vi "RIOTargetUI.vi"() -> ()   [LabVIEW 2014, in "RIO Target.lvclass"]
doc: "UI that will be called when the node is selected."
uses:
  RIO Target/RIO Target.lvclass
  <vilib>/NI/Configuration Framework/Node/NodeRef.ctl
  <vilib>/NI/Configuration Framework/Node/NISE_CEF_Node.lvclass
  <vilib>/NI/AMC/Message Queue.ctl
  <vilib>/NI/AMC/Message.ctl
  <vilib>/NI/Tools/Keyed Array/KeyedArray.ctl
  <vilib>/NI/Configuration Framework/Node/UserEventRef.ctl
  <vilib>/NI/Configuration Framework/Controls/EventCluster.ctl
  RIO Target/RIO Target.lvclass/RIO Target.ctl
  RIO Target Configuration/RIO Target Configuration.lvclass/RIO Target Configuration.ctl
  RIO Target Configuration/RIO Target Configuration.lvclass
  <vilib>/NI/Configuration Framework/serializable configuration/NISE_CEF_serializable configuration.lvclass
  <vilib>/NI/Tools/Keyed Array/Tools_KeyedArray.lvlib
  <vilib>/NI/AMC/AMC.lvlib
  <vilib>/NI/Configuration Framework/NISE_CEF_TreeControl.lvlib
panel:
  in  "CLIP XML Path":path
  in  "Use Custom CLIP?":bool
  out "Number of Channels":u32
  out "Number of Devices":u32
  out "Number of Buses":u32
  out "Channels per Device":string[][](table)
  in  "Target Destination VI":path
  in  "Replace Default Destination VI?":bool
  in  "Target Project Path":path
  in  "Comments":string
  in  "Alias":string
  in  "user event":T1
  in  "main queue":T2
  in  "node ref":T3
  # "Settings"
  # "Target Destination VI"
  # "CLIP XML Path"
  # "Target Summary"
  # "Number of Buses"
  # "Number of Devices"
  # "Number of Channels"
  # "Channels per Device"
  # "Target Project Path"
  # "Comments"
  # "Alias"
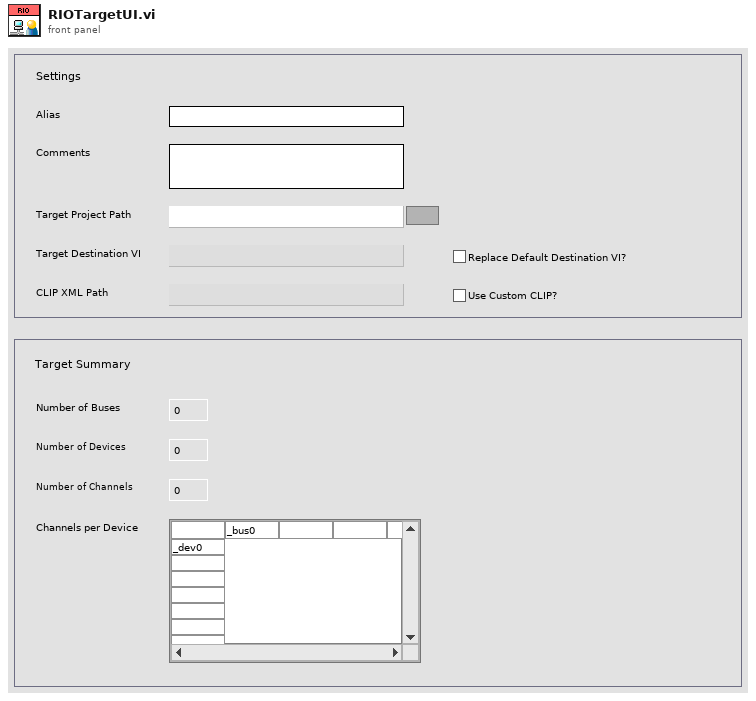
[diagram p1: front panel]
types:
  T1 = typedef "NISE_CEF_Node.lvclass/UserEventRef.ctl" = refnum<user-event>
  T2 = typedef "AMC.lvlib/Message Queue.ctl" = refnum<queue>
  T3 = typedef "NISE_CEF_Node.lvclass/NodeRef.ctl" = refnum<data-value>
  T4 = typedef "RIO Target.lvclass/UI Configuration.ctl" = cluster{"Destination VI":path, "Target Project Path":path, "CLIP XML Path":path, "Alias":string, "Comments":string, "Replace Default VI?":bool, "Use Custom CLIP?":bool}
  T5 = enum8{"Enabled", "Disabled", "Disabled and Grayed Out"}
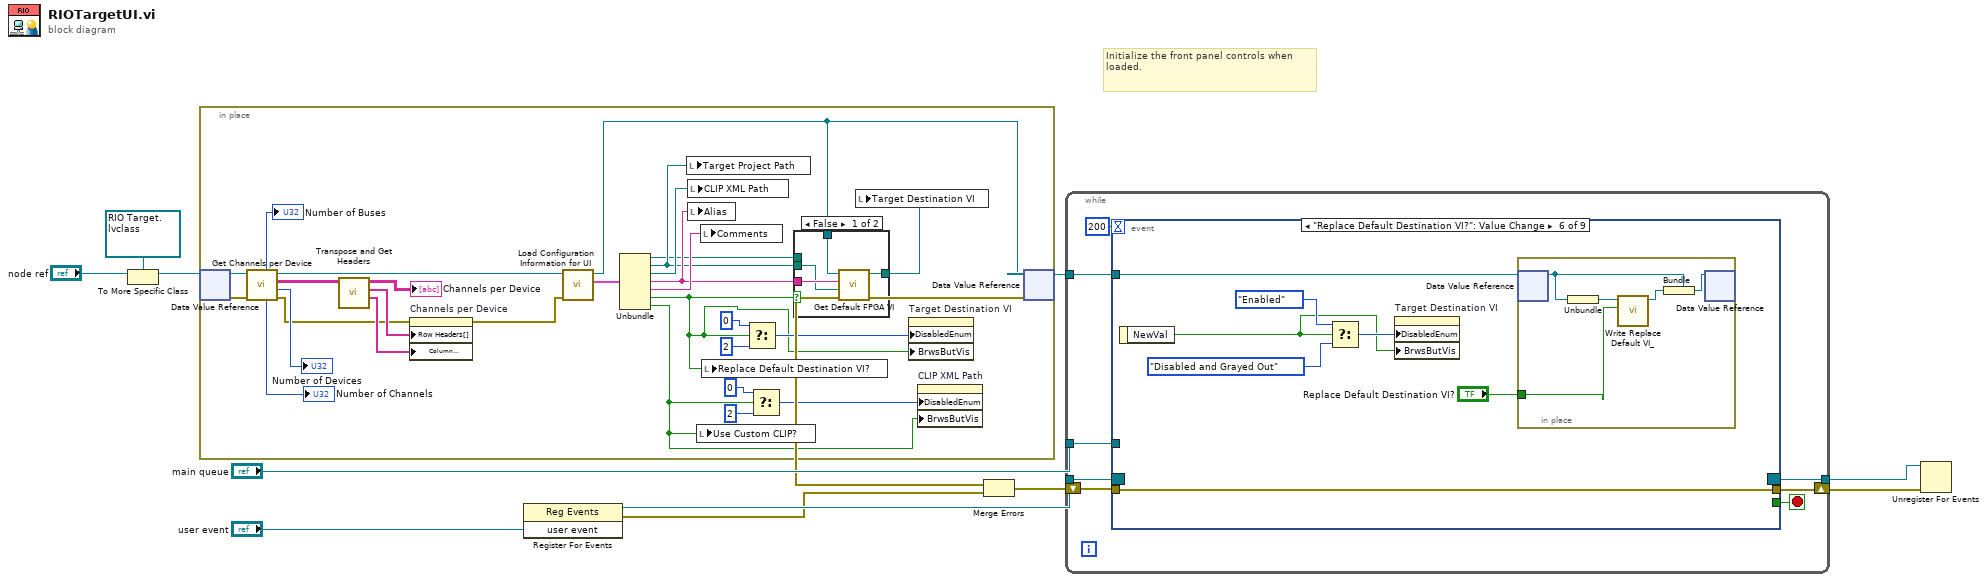
[diagram p0: block diagram]
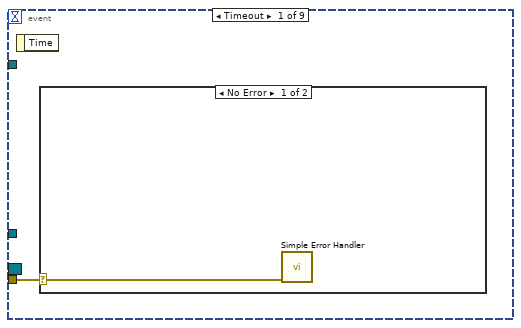
[diagram p2: hidden frame]
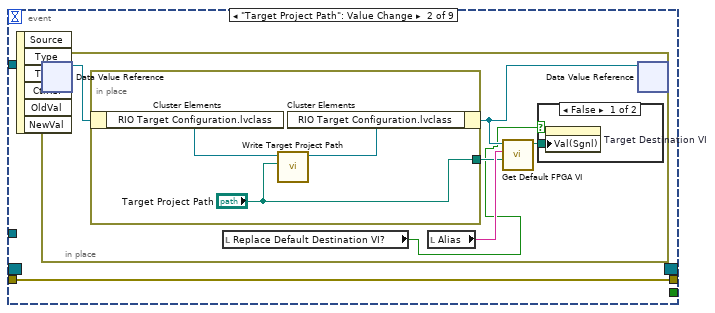
[diagram p4: hidden frame]
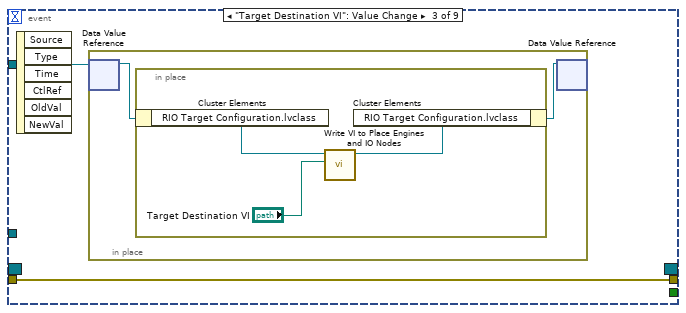
[diagram p6: hidden frame]
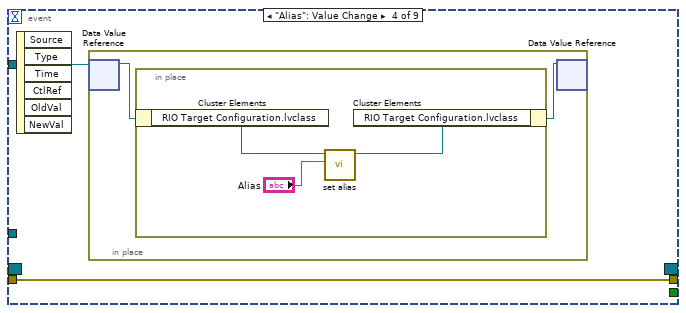
[diagram p7: hidden frame]
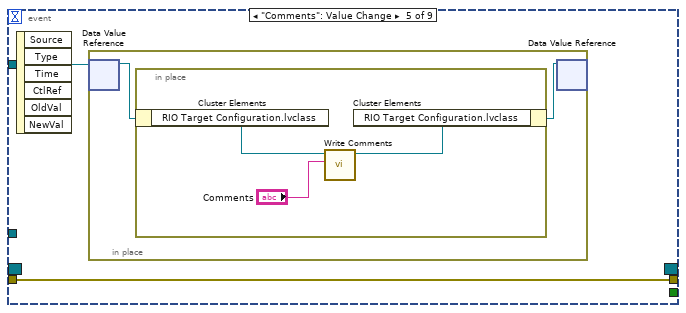
[diagram p8: hidden frame]
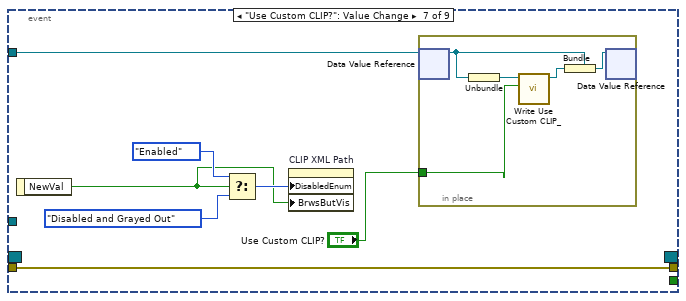
[diagram p9: hidden frame]
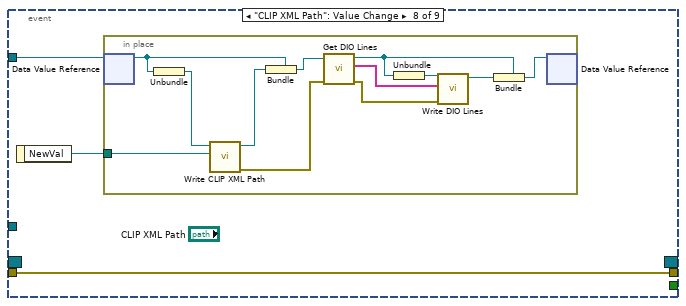
[diagram p10: hidden frame]
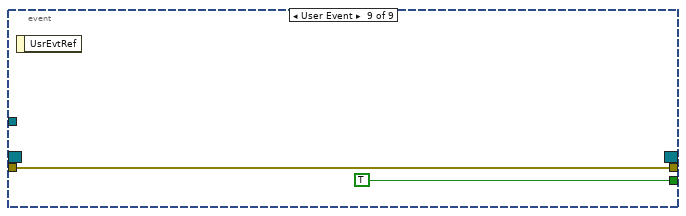
[diagram p11: hidden frame]
diagram:
  # "Initialize the front panel controls when loaded."
  n1 = To More Specific Class(target class=refnum<data-value> refnum ("data value reference"), reference="node ref") -> (specific class reference=w2:refnum<data-value>)  [unwired: 1 in, 1 out]
  n2 = in-place {
    n3 = in-place-dvr #1(w2) -> (w40:refnum<class "RIO Target.lvclass">, w39:errorcluster)
    n4 = call "Get Channels per Device.vi"("error in (no error)"=w39, "RIO Target in"=w40) -> ("error out"=w31:errorcluster, "Number of Devices"=→"Number of Devices":i32, "Channels per Device"=w35:string[][], "RIO Target out"=w30:refnum<class "RIO Target.lvclass">, "Number of Channels"=→"Number of Channels":u32, "Number of Buses"=→"Number of Buses":i32)  [unwired: 4 in]
    n5 = call "Transpose and Get Headers.vi"("Channels per Device'"=w35) -> ("Column Headers"=w32:string[], "Row Headers"=w33:string[], "Channels per Device"=→"Channels per Device":string[][])  [unwired: 8 in]
    n6 = property on="Channels per Device" class="Tbl (strict)"(error in=w31, "Row Headers[]"=w33, "Column Headers[]"=w32) -> (error out=w29:errorcluster)  [unwired: 1 in, 1 out]
    n7 = call "Load Configuration Information for UI.vi"("error in (no error)"=w29, "node in"=w30) -> ("UI Configuration"=w28:T4, "node out"=w15:refnum<class "RIO Target.lvclass">)  [unwired: 7 in, 1 out]
    n8 = Unbundle(w28) -> ("Destination VI"=w23:path, "Target Project Path"=w24:path, "CLIP XML Path"=w27:path, "Alias"=w25:string, "Comments"=w26:string, "Replace Default VI?"=w16:bool, "Use Custom CLIP?"=w13:bool)
    n9 = local write "Target Project Path"(w24) -> ()
    n10 = local write "CLIP XML Path"(w27) -> ()
    n11 = local write "Alias"(w25) -> ()
    n12 = local write "Use Custom CLIP?"(w13) -> ()
    n13 = local write "Comments"(w26) -> ()
    n14 = local write "Replace Default Destination VI?"(w16) -> ()
    n15 = Select(t=0, s=w16, f=2) -> (s? t:f=w18:i32)
    n16 = Select(t=0, s=w13, f=2) -> (s? t:f=w17:i32)
    n17 = case shown="False" w16 {
      tunnel: w15 -> [w44 _]
      tunnel: w25 -> [w43 _]
      tunnel: w24 -> [w42 _]
      tunnel: [w41 w45] -> w22
      tunnel: w23 -> [_ w45]
      frame False {
        n18 = call "Get Default FPGA VI.vi"("Target Project Path"=w42, "Alias"=w43, "LabVIEW Object in"=w44) -> ("appended path"=w41:path)  [unwired: 8 in]
      }
      frame True {
      }
    }
    n19 = local write "Target Destination VI"(w22) -> ()
    n20 = property on="Target Destination VI" class="Path"("DisabledEnum"=w18, "BrwsButVis"=w16) -> ()  [unwired: 2 in, 2 out]
    n21 = property on="CLIP XML Path" class="Path"("DisabledEnum"=w17, "BrwsButVis"=w13) -> ()  [unwired: 2 in, 2 out]
    n22 = in-place-dvr #1(w15) -> (w12:refnum<data-value>, w6:errorcluster)
  }
  n23 = register-events("user event") -> (reference out=w9:refnum<event-registration>, error out=w1:errorcluster)  [unwired: 2 in]
  n24 = Merge Errors(w6, w1) -> (w5:errorcluster)
  n25 = while {
    tunnel: w12 -> [w53]
    tunnel: "main queue" -> [w52]
    tunnel: w9 -> [w50]
    tunnel: [w49] -> w8
    shift-right: [w47] -> w7
    shift-left: w5 -> [w46]
    stop <- w48 stop-if-true
    n26 = event shown="[5] \"Replace Default Destination VI?\": Value Change" {
      selector: w50 -> [_ _ _ _ _ _ _ _ _]
      dyn-events: [_ _ _ _ _ _ _ _ _] -> w49
      timeout: 200 -> [_ _ _ _ _ _ _ _ _]
      tunnel: w53 -> [_ w56 w68 w75 w82 w90 w102 w114 _]
      tunnel: w52 -> [_ _ _ _ _ _ _ _ _]
      tunnel: [_ _ _ _ _ _ _ _ TRUE] -> w48
      tunnel: [_ w57 w69 w76 w83 w95 w107 w115 w128] -> w47
      tunnel: w46 -> [w54 w57 w69 w76 w83 w95 w107 w115 w128]
      event Timeout {
        n27 = event-data() -> ()  [unwired: 1 in, 1 out]
        n28 = case shown="No Error" w54 {
          selector: w54 -> [w55 _]
          frame No Error {
            n29 = call <vilib>:"Simple Error Handler.vi"("error in (no error)"=w55) -> ()  [unwired: 4 in, 5 out]
          }
          frame Error {
          }
        }
      }
      event "Target Project Path": Value Change {
        n30 = event-data() -> ()  [unwired: 1 in, 6 out]
        n31 = in-place {
          n32 = in-place-dvr #2(w56) -> (w63:refnum<class "RIO Target.lvclass">)  [unwired: 1 out]
          n33 = in-place {
            in-place-border: ["Target Project Path"] -> w59
            n34 = in-place-cluster #3(w63) -> ("RIO Target Configuration.lvclass"=w67:refnum<class "RIO Target Configuration.lvclass">)
            n35 = call "Write Target Project Path.vi"("Target Project Path"="Target Project Path", "RIO Target Configuration in"=w67) -> ("RIO Target Configuration out"=w66:refnum<class "RIO Target Configuration.lvclass">)  [unwired: 8 in, 1 out]
            n36 = in-place-cluster #3("RIO Target Configuration.lvclass"=w66) -> (w62:refnum<class "RIO Target.lvclass">)
          }
          n37 = local read "Replace Default Destination VI?"() -> (w58:bool)
          n38 = local read "Alias"() -> (w61:string)
          n39 = call "Get Default FPGA VI.vi"("Target Project Path"=w59, "Alias"=w61, "LabVIEW Object in"=w62) -> ("appended path"=w60:path)  [unwired: 8 in]
          n40 = case shown="False" w58 {
            tunnel: w60 -> [w64 _]
            frame False {
              n41 = property on="Target Destination VI" class="Path"("Val(Sgnl)"=w64) -> ()  [unwired: 2 in, 2 out]
            }
            frame True {
            }
          }
          n42 = in-place-dvr #2(w62) -> ()  [unwired: 2 out]
        }
      }
      event "Target Destination VI": Value Change {
        n43 = event-data() -> ()  [unwired: 1 in, 6 out]
        n44 = in-place {
          n45 = in-place-dvr #4(w68) -> (w71:refnum<class "RIO Target.lvclass">)  [unwired: 1 out]
          n46 = in-place {
            n47 = in-place-cluster #5(w71) -> ("RIO Target Configuration.lvclass"=w74:refnum<class "RIO Target Configuration.lvclass">)
            n48 = call "Write VI to Place Engines and IO Nodes.vi"("VI to Place Engines and IO Nodes"="Target Destination VI", "RIO Target Configuration in"=w74) -> ("RIO Target Configuration out"=w73:refnum<class "RIO Target Configuration.lvclass">)  [unwired: 8 in, 1 out]
            n49 = in-place-cluster #5("RIO Target Configuration.lvclass"=w73) -> (w70:refnum<class "RIO Target.lvclass">)
          }
          n50 = in-place-dvr #4(w70) -> ()  [unwired: 2 out]
        }
      }
      event "Alias": Value Change {
        n51 = event-data() -> ()  [unwired: 1 in, 6 out]
        n52 = in-place {
          n53 = in-place-dvr #6(w75) -> (w78:refnum<class "RIO Target.lvclass">)  [unwired: 1 out]
          n54 = in-place {
            n55 = in-place-cluster #7(w78) -> ("RIO Target Configuration.lvclass"=w81:refnum<class "RIO Target Configuration.lvclass">)
            n56 = call <vilib>:"set alias.vi"("alias"="Alias", "configuration in"=w81) -> ("configuration out"=w80:refnum<class "RIO Target Configuration.lvclass">)  [unwired: 8 in, 1 out]
            n57 = in-place-cluster #7("RIO Target Configuration.lvclass"=w80) -> (w77:refnum<class "RIO Target.lvclass">)
          }
          n58 = in-place-dvr #6(w77) -> ()  [unwired: 2 out]
        }
      }
      event "Comments": Value Change {
        n59 = event-data() -> ()  [unwired: 1 in, 6 out]
        n60 = in-place {
          n61 = in-place-dvr #8(w82) -> (w85:refnum<class "RIO Target.lvclass">)  [unwired: 1 out]
          n62 = in-place {
            n63 = in-place-cluster #9(w85) -> ("RIO Target Configuration.lvclass"=w88:refnum<class "RIO Target Configuration.lvclass">)
            n64 = call "Write Comments.vi"("Comments"="Comments", "RIO Target Configuration in"=w88) -> ("RIO Target Configuration out"=w87:refnum<class "RIO Target Configuration.lvclass">)  [unwired: 8 in, 1 out]
            n65 = in-place-cluster #9("RIO Target Configuration.lvclass"=w87) -> (w84:refnum<class "RIO Target.lvclass">)
          }
          n66 = in-place-dvr #8(w84) -> ()  [unwired: 2 out]
        }
      }
      event "Replace Default Destination VI?": Value Change {
        n67 = event-data() -> ("NewVal"=w91:bool)  [unwired: 1 in]
        n68 = Select(t=T5."Enabled" ("Disabled"), s=w91, f=T5."Disabled and Grayed Out" ("Disabled")) -> (s? t:f=w92:T5)
        n69 = property on="Target Destination VI" class="Path"("DisabledEnum"=w92, "BrwsButVis"=w91) -> ()  [unwired: 2 in, 2 out]
        n70 = in-place {
          in-place-border: "Replace Default Destination VI?" -> [w99]
          n71 = in-place-dvr #10(w90) -> (w97:refnum<class "RIO Target.lvclass">)  [unwired: 1 out]
          n72 = Unbundle(w97) -> (w100:refnum<class "RIO Target Configuration.lvclass">)
          n73 = call "Write Replace Default VI_.vi"("Replace Default VI?"=w99, "RIO Target Configuration in"=w100) -> ("RIO Target Configuration out"=w98:refnum<class "RIO Target Configuration.lvclass">)  [unwired: 8 in, 1 out]
          n74 = Bundle(cluster=w97, w98) -> (w96:refnum<class "RIO Target.lvclass">)
          n75 = in-place-dvr #10(w96) -> ()  [unwired: 2 out]
        }
      }
      event "Use Custom CLIP?": Value Change {
        n76 = event-data() -> ("NewVal"=w103:bool)  [unwired: 1 in]
        n77 = Select(t=T5."Enabled" ("Disabled"), s=w103, f=T5."Disabled and Grayed Out" ("Disabled")) -> (s? t:f=w104:T5)
        n78 = property on="CLIP XML Path" class="Path"("DisabledEnum"=w104, "BrwsButVis"=w103) -> ()  [unwired: 2 in, 2 out]
        n79 = in-place {
          in-place-border: "Use Custom CLIP?" -> [w111]
          n80 = in-place-dvr #11(w102) -> (w109:refnum<class "RIO Target.lvclass">)  [unwired: 1 out]
          n81 = Unbundle(w109) -> (w112:refnum<class "RIO Target Configuration.lvclass">)
          n82 = call "Write Use Custom CLIP_.vi"("Use Custom CLIP?"=w111, "RIO Target Configuration in"=w112) -> ("RIO Target Configuration out"=w110:refnum<class "RIO Target Configuration.lvclass">)  [unwired: 8 in, 1 out]
          n83 = Bundle(cluster=w109, w110) -> (w108:refnum<class "RIO Target.lvclass">)
          n84 = in-place-dvr #11(w108) -> ()  [unwired: 2 out]
        }
      }
      event "CLIP XML Path": Value Change {
        n85 = event-data() -> ("NewVal"=w113:path)  [unwired: 1 in]
        n86 = in-place {
          in-place-border: w113 -> [w127]
          n87 = in-place-dvr #12(w114) -> (w124:refnum<class "RIO Target.lvclass">)  [unwired: 1 out]
          n88 = Unbundle(w124) -> (w125:refnum<class "RIO Target Configuration.lvclass">)
          n89 = call "Write CLIP XML Path.vi"("CLIP XML Path"=w127, "RIO Target Configuration in"=w125) -> ("error out"=w126:errorcluster, "RIO Target Configuration out"=w123:refnum<class "RIO Target Configuration.lvclass">)  [unwired: 8 in]
          n90 = Bundle(cluster=w124, w123) -> (w122:refnum<class "RIO Target.lvclass">)
          n91 = call "Get DIO Lines.vi"("error in (no error)"=w126, "RIO Target in"=w122) -> ("error out"=w119:errorcluster, "DIO Lines"=w120:string[], "RIO Target out"=w117:refnum<class "RIO Target.lvclass">)  [unwired: 7 in]
          n92 = Unbundle(w117) -> (w121:refnum<class "RIO Target Configuration.lvclass">)
          n93 = call "Write DIO Lines.vi"("error in (no error)"=w119, "DIO Lines"=w120, "RIO Target Configuration in"=w121) -> ("RIO Target Configuration out"=w118:refnum<class "RIO Target Configuration.lvclass">)  [unwired: 7 in, 1 out]
          n94 = Bundle(cluster=w117, w118) -> (w116:refnum<class "RIO Target.lvclass">)
          n95 = in-place-dvr #12(w116) -> ()  [unwired: 2 out]
        }
      }
      event User Event {
        n96 = event-data() -> ()  [unwired: 1 in, 1 out]
      }
    }
  }
  n97 = Unregister For Events(event registration refnum=w8, error in=w7) -> ()  [unwired: 1 out]
